vi "AdvServoOpen.vi"(8 "error in":errorcluster, 9 "milliseconds":i32=5000, 10 "Serial Number":i32=-1, 11 "Device In":i32) -> (0 "error out":errorcluster, 1 "Attached?":bool, 2 "Serial Number Return":i32, 3 "Device Out":i32)   [LabVIEW 2014]
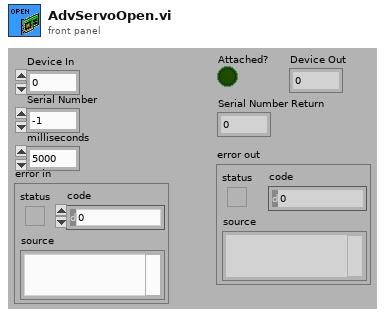
[diagram p1: front panel]
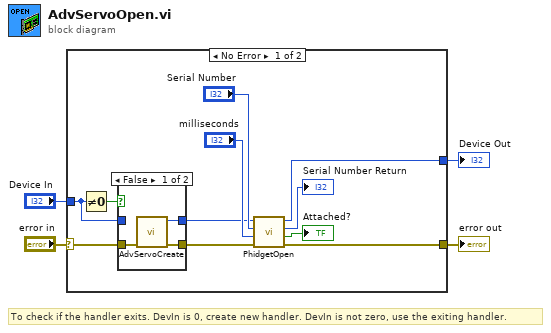
[diagram p0: block diagram]
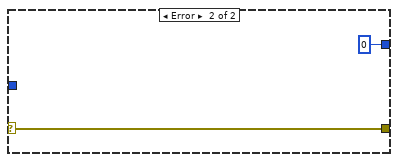
[diagram p3: hidden frame]
diagram:
  # "To check if the handler exits. DevIn is 0, create new handler. DevIn is not zero, use the exiting handler."
  n1 = case shown="No Error" "error in" {
    selector: "error in" -> [w15 w22]
    tunnel: [w7 w22] -> w3
    tunnel: [w8 0 ("return type")] -> w2
    tunnel: "Device In" -> [w10 _]
    frame No Error {
      n2 = Not Equal To 0?(x=w10) -> (x != 0?=w11:bool)
      n3 = case shown="False" w11 {
        tunnel: w15 -> [w16 w19]
        tunnel: [w17 w19] -> w14
        tunnel: [w18 w20] -> w9
        tunnel: w10 -> [_ w20]
        frame False {
          n4 = call "AdvServoCreate.vi"("error in"=w16) -> ("error out"=w17:errorcluster, "Device Out"=w18:i32)  [unwired: 9 in]
        }
        frame True {
        }
      }
      n5 = call "PhidgetOpen.vi"("error in"=w14, "milliseconds"="milliseconds", "Serial Number"="Serial Number", "Device In"=w9) -> ("error out"=w7:errorcluster, "Attached?"=→"Attached?":bool, "Serial Number Return"=→"Serial Number Return":i32, "Device Out"=w8:i32)  [unwired: 4 in]
    }
    frame Error {
    }
  }
  "error out" <- w3
  "Device Out" <- w2
